vi "Close Laser AO.vi"(8 "error in":errorcluster, 11 "cPAS in":refnum<class "cPAS.lvclass">) -> (0 "error out":errorcluster, 3 "cPAS out":refnum<class "cPAS.lvclass">)   [LabVIEW 2015, in "cPAS.lvclass"]
uses:
  cPAS.lvclass
  cPAS.lvclass/cPAS.ctl
  <vilib>/Utility/error.llb/Error Cluster From Error Code.vi
  <vilib>/rvi/errors/niLvFpgaAdjustHostInterfaceError.vi
  <vilib>/FPGAPlugInAG/PXI-7841R/niLvFpga_Close_PXI-7841R.vi
  <vilib>/rvi/interface/nirviReadWriteControl/nirviReadWriteControl.xnode
  Interface/fpga_ctl.ctl
  FPGA Bitfiles/FPGA Server.lvbitx
  <vilib>/rvi/interface/nirviCloseFPGA/nirviCloseFPGA.xnode
  NiFpgaLv.dll
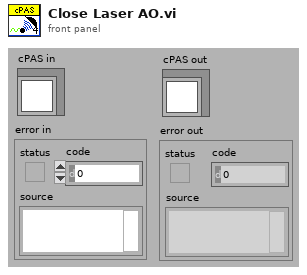
[diagram p1: front panel]
types:
  T1 = typedef "fpga_ctl.ctl" = refnum<k20>
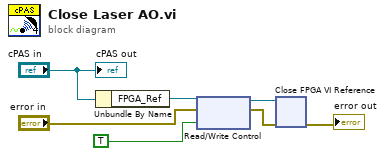
[diagram p0: block diagram]
diagram:
  n1 = Unbundle By Name("cPAS in") -> ("FPGA_Ref"=w4:T1)
  n2 = xnode "Read/Write Control"("FPGA VI Reference In"=w4, "error in"="error in", "stop"=TRUE) -> ("FPGA VI Reference Out"=w5:T1, "error out"=w7:errorcluster)
  n3 = xnode "Close FPGA VI Reference"("FPGA VI Reference In"=w5, "error in"=w7) -> ("error out"=→"error out":errorcluster)
  "cPAS out" <- "cPAS in"
